vi "UDP1_packet_speed (SubVI).vi"(11 "Data_size":i32) -> (3 "UDP1_packet_speed":dbl)   [LabVIEW 2017]
uses:
  Global_SNK3_HF.vi
panel:
  out "x .or. y?":bool
  out "millisecond timer value":u32
  out "timer_start_meas":u32
  in  "Total_data_size":i32
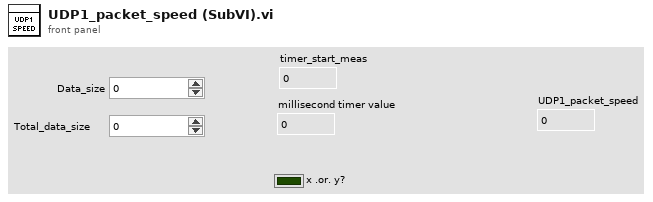
[diagram p1: front panel]
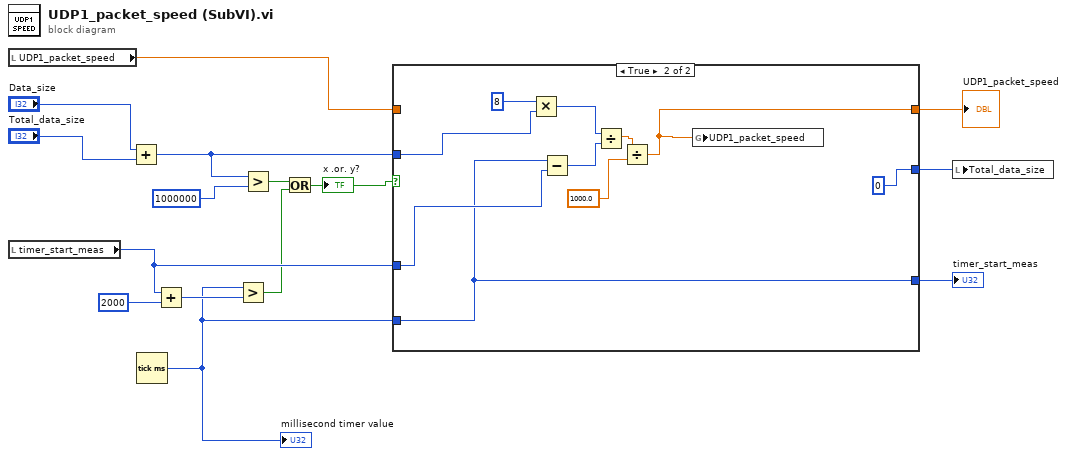
[diagram p0: block diagram]
diagram:
  n1 = local read "UDP1_packet_speed"() -> (w3:dbl)
  n2 = local read "timer_start_meas"() -> (w8:u32)
  n3 = Add(x="Data_size", y="Total_data_size") -> (x+y=w11:i32)
  n4 = Tick Count (ms)() -> (millisecond timer value=w1:u32)
  "millisecond timer value" <- w1
  n5 = Add(x=w8, y=u32 2000) -> (x+y=w2:u32)
  n6 = Greater?(x=w1, y=w2) -> (0:w6:bool)
  n7 = Greater?(x=w11, y=1000000) -> (0:w7:bool)
  n8 = Or(x=w7, y=w6) -> (x .or. y?=w5:bool)
  "x .or. y?" <- w5
  n9 = case shown="True" w5 {
    tunnel: [w18 0 ("Total_data_size")] -> w12
    tunnel: w11 -> [w18 w24]
    tunnel: w8 -> [w17 w27]
    tunnel: [w17 w25] -> w10
    tunnel: w1 -> [_ w25]
    tunnel: [w16 w19] -> w4
    tunnel: w3 -> [w16 _]
    frame False {
    }
    frame True {
      n10 = Multiply(x=8, y=w24) -> (x*y=w22:i32)
      n11 = Subtract(x=w25, y=w27) -> (x-y=w26:u32)
      n12 = Divide(x=w22, y=w26) -> (x/y=w21:dbl)
      n13 = Divide(x=w21, y=1000.0) -> (x/y=w19:dbl)
      n14 = global write "Global_SNK3_HF.vi" "UDP1_packet_speed"(w19) -> ()
    }
  }
  "timer_start_meas" <- w10
  "UDP1_packet_speed" <- w4
  n15 = local write "Total_data_size"(w12) -> ()
